vi "Actor Core.vi"(8 "error in":errorcluster, 11 "Basic Demo in":refnum<class "Basic Demo.lvclass">) -> (0 "error out":errorcluster, 3 "Actor out":refnum<class "Actor.lvclass">)   [LabVIEW 2020, in "2. Basic Panel Actors.lvlib" / "Basic Demo.lvclass"]
doc: "Allows the user to launch more panels of different types.\n----\nCopyright: MGI 2016\nAuthor: Derek Trepanier"
uses:
  Basic Demo.lvclass
  C:/Program Files/National Instruments/LabVIEW 2020/vi.lib/MGI/Panel Manager/Panel Actor/Panel Actor/Panel Actor.lvclass
  <vilib>/ActorFramework/Actor/Actor.lvclass
  Panel/Sample Panel.lvclass
  <vilib>/ActorFramework/Message Enqueuer/Message Enqueuer.lvclass
  <vilib>/ActorFramework/Message Enqueuer/Message Enqueuer.lvclass/Message Enqueuer.ctl
  <vilib>/ActorFramework/Message Enqueuer/Enqueue.vi
  Description Panel/Description Panel.lvclass
  <vilib>/MGI/Panel Manager/Panel/Panel/Subpanel/Subpanel.lvclass
  C:/Program Files/National Instruments/LabVIEW 2020/vi.lib/MGI/Panel Manager/Panel/Panel/Panel.lvclass
  <vilib>/ActorFramework/Stop Msg/Stop Msg.lvclass
  C:/Program Files/National Instruments/LabVIEW 2020/vi.lib/ActorFramework/Message/Message.lvclass
  <vilib>/MGI/Panel Manager/Panel/Panel/Window/Dialog/Dialog.lvclass
  <vilib>/MGI/Panel Manager/Panel/Panel/Window/Window.lvclass
  <vilib>/MGI/Panel Manager/Panel/Panel/Subpanel/Subpanel.vi
  <vilib>/ActorFramework/Message Priority Queue/Priority Enqueue.vi
  <vilib>/MGI/Panel Manager/Panel/Panel/Window/Dialog/Dialog.vi
  <vilib>/MGI/Panel Manager/Panel/Panel/Window/Window.vi
  <vilib>/MGI/Panel Manager/Panel Actor/Panel Actor/Panel Actor.lvclass
  <vilib>/MGI/Panel Manager/Panel Actor/Panel Actor Messages/Show Panel Msg/Show Panel Msg.lvclass
  <vilib>/MGI/Panel Manager/Panel/Panel.lvlib
panel:
  in  "Show Window":bool
  in  "Show Dialog":bool
  in  "Running Sub-Panels":i32(listbox)
  in  "New Subpanel Item":bool
  # "Windows"
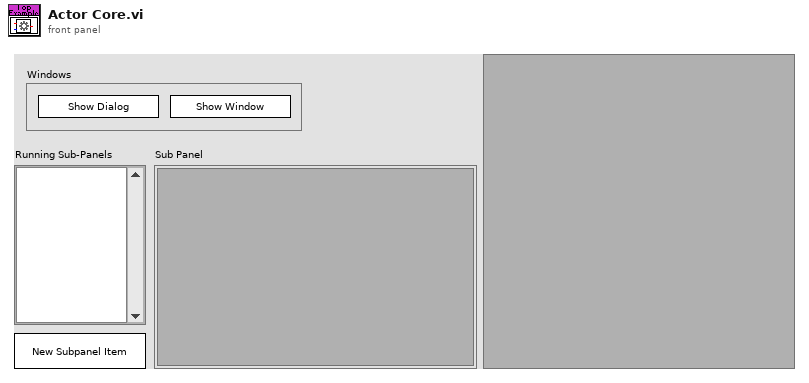
[diagram p1: front panel]
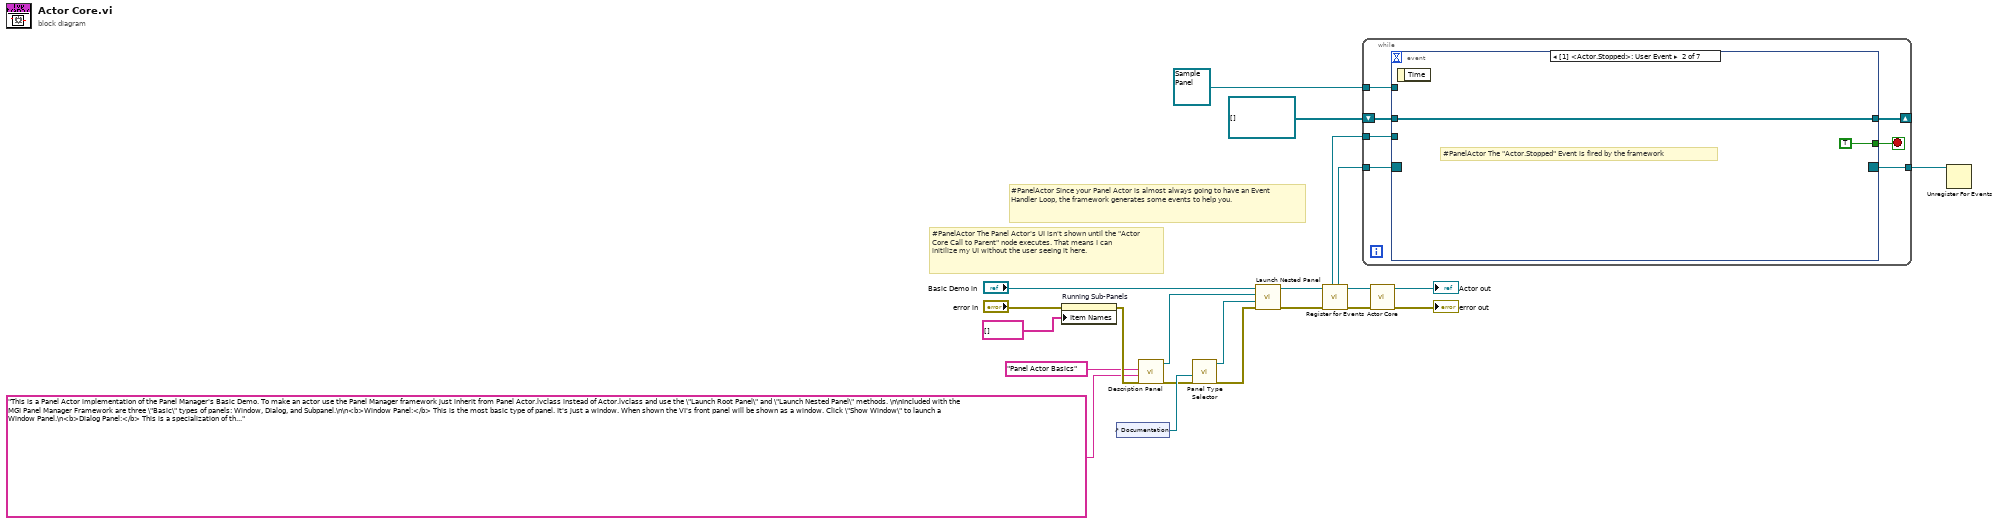
[diagram p0: block diagram]
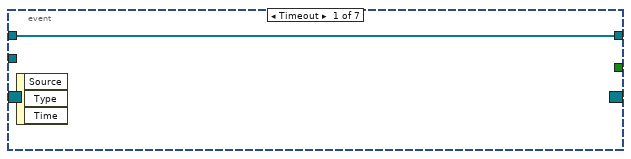
[diagram p2: hidden frame]
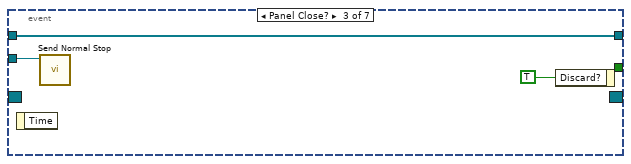
[diagram p3: hidden frame]
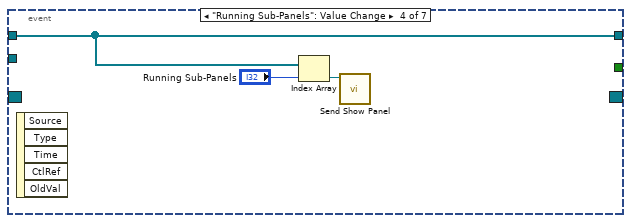
[diagram p4: hidden frame]
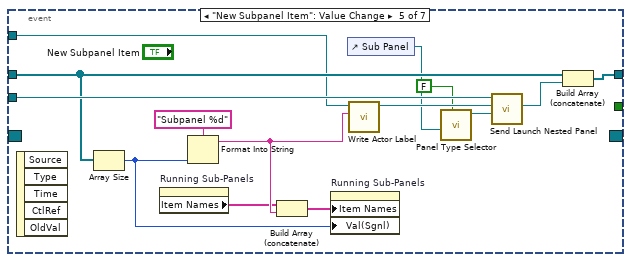
[diagram p5: hidden frame]
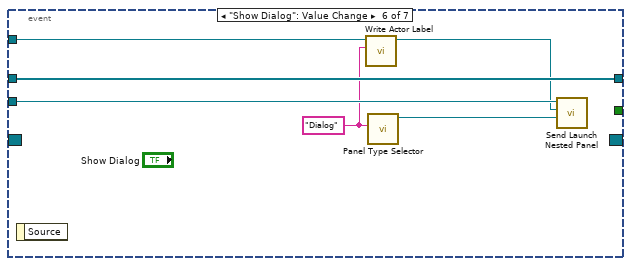
[diagram p6: hidden frame]
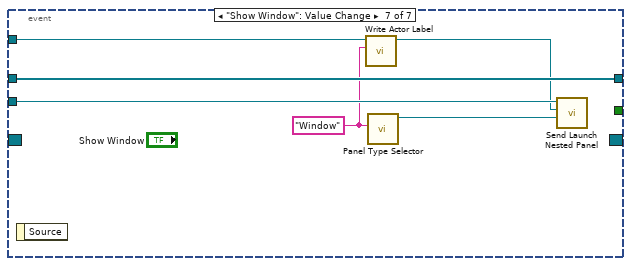
[diagram p7: hidden frame]
diagram:
  # "#PanelActor Since your Panel Actor is almost always going to have an Event Handler Loop, the framework generates some events to help you."
  # "#PanelActor The Panel Actor's UI isn't shown until the \"Actor Core Call to Parent\" node executes. That means I can initilize my UI without the user seeing it here."
  n1 = property on="Running Sub-Panels" class="LstBox (strict)"(error in="error in", "Item Names"=string[] []) -> (error out=w8:errorcluster)  [unwired: 1 in, 1 out]
  n2 = control-ref of="Documentation"() -> (w16:refnum<vi>)
  n3 = call "Description Panel.vi"("error in (no error)"=w8, "Description"="This is a Panel Actor implementation of the Panel Manager's Basic Demo. To make an actor use the Panel Manager framework just inherit from Panel Actor.lvclass instead of Actor.lvclass and use the \"Launch Root Panel\" and \"Launch Nested Panel\" methods. \n\nIncluded with the MGI Panel Manager Framework are three \"Basic\" types of panels: Window, Dialog, and Subpanel.\n\n<b>Window Panel:</b> This is the most basic type of panel. It's just a window. When shown the VI's front panel will be shown as a window. Click \"Show Window\" to launch a Window Panel.\n<b>Dialog Panel:</b> This is a specialization of the window panel. Again, the window will just be shown as a window, but the front panel will be set to modal. Click \"Show Dialog\" to launch a Dialog Panel.\n<b>Subpanel:</b> This panel type will insert the front panel into a subpanel of another VI. Click \"New Subpanel Item\" to launch a new Subpanel Panel. The list of running subpanel items is show in the \"Running Sub-Panels\" \n\nView the #PanelActor bookmark for more info.\n" ("Description Title"), "Description Title"="Panel Actor Basics") -> ("error out"=w7:errorcluster, "Description Panel out"=w4:refnum<class "Description Panel.lvclass">)  [unwired: 7 in]
  n4 = call-poly <vilib>:"Panel Type Selector.vi"("Error In"=w7, "Sub Panel"=w16) -> ("Error Out"=w6:errorcluster, "Subpanel Out"=w5:refnum<class "Subpanel.lvclass">)  [unwired: 8 in]
  n5 = call <vilib>:"Launch Nested Panel.vi"("error in (no error)"=w6, "Panel"=w5, "Nested Panel Actor"=w4, "Panel Actor in"="Basic Demo in") -> ("error out"=w9:errorcluster, "Panel Actor out"=w10:refnum<class "Basic Demo.lvclass">)  [unwired: 4 in, 2 out]
  n6 = call <vilib>:"Register for Events.vi"("Error In"=w9, "Panel Actor in"=w10) -> ("Error Out"=w20:errorcluster, "Panel Actor out"=w21:refnum<class "Basic Demo.lvclass">, "Pnl Actor"=w19:refnum<event-registration>, "Self Enqueuer"=w18:refnum<class "Message Enqueuer.lvclass">)  [unwired: 6 in]
  n7 = while {
    tunnel: w19 -> [w29]
    tunnel: w18 -> [w28]
    shift-right: [w25] -> _
    shift-left: refnum<class "Message Enqueuer.lvclass">[] [] -> [w26]
    tunnel: refnum<class "Sample Panel.lvclass"> refnum ("Basic Panel Actors.lvlib:Panel.lvclass") -> [w24]
    tunnel: [w23] -> w1
    stop <- w27 stop-if-true
    n8 = event shown="[1] <Actor.Stopped>: User Event" {
      selector: w29 -> [_ _ _ _ _ _ _]
      dyn-events: [_ _ _ _ _ _ _] -> w23
      timeout: _ -> [_ _ _ _ _ _ _]
      tunnel: w28 -> [_ _ w34 _ w49 w57 w63]
      tunnel: [_ TRUE _ _ _ _ _] -> w27
      tunnel: w26 -> [w30 w31 w33 w38 w46 w58 w64]
      tunnel: [w30 w31 w33 w38 w52 w58 w64] -> w25
      tunnel: w24 -> [_ _ _ _ w44 w56 w62]
      event Timeout {
        n9 = event-data() -> ()  [unwired: 1 in, 3 out]
      }
      event User Event {
        # "#PanelActor The \"Actor.Stopped\" Event is fired by the framework"
        n10 = event-data() -> ()  [unwired: 1 in, 1 out]
      }
      event Panel Close? {
        n11 = event-data() -> ()  [unwired: 1 in, 1 out]
        n12 = call <vilib>:"Send Normal Stop.vi"("Message Enqueuer"=w34) -> ()  [unwired: 10 in, 1 out]
        n13 = event-data("Discard?"=TRUE) -> ()  [unwired: 1 in, 1 out]
      }
      event "Running Sub-Panels": Value Change {
        n14 = event-data() -> ()  [unwired: 1 in, 5 out]
        n15 = Index Array(array=w38, index="Running Sub-Panels") -> (element=w37:refnum<class "Message Enqueuer.lvclass">)
        n16 = call <vilib>:"Send Show Panel.vi"("Message Enqueuer in"=w37) -> ()  [unwired: 9 in, 2 out]
      }
      event "New Subpanel Item": Value Change {
        n17 = event-data() -> ()  [unwired: 1 in, 5 out]
        n18 = Array Size(array=w46) -> (size(s)=w41:i32)
        n19 = property on="Running Sub-Panels" class="LstBox (strict)"() -> ("Item Names"=w43:string[])  [unwired: 2 in, 2 out]
        n20 = Format Into String(format string="Subpanel %d", w41) -> (resulting string=w45:string)  [unwired: 2 in, 1 out]
        n21 = Build Array (concatenate)(w43, w45) -> (w42:string[])
        n22 = property on="Running Sub-Panels" class="LstBox (strict)"("Item Names"=w42, "Val(Sgnl)"=w41) -> ()  [unwired: 2 in, 2 out]
        n23 = control-ref of="Sub Panel"() -> (w40:refnum<vi>)
        n24 = call-dynamic "Write Actor Label.vi"("Actor Label"=w45, "Monitored Actor in"=w44) -> ("Monitored Actor out"=w48:refnum<class "Sample Panel.lvclass">)  [unwired: 8 in, 1 out]
        n25 = call-poly <vilib>:"Panel Type Selector.vi"("Autoshow? (T)"=FALSE, "Sub Panel"=w40) -> ("Subpanel Out"=w50:refnum<class "Subpanel.lvclass">)  [unwired: 8 in, 1 out]
        n26 = call <vilib>:"Send Launch Nested Panel.vi"("Panel"=w50, "Nested Panel Actor"=w48, "Self Enqueuer in"=w49) -> ("Nested Actor's Enqueuer"=w51:refnum<class "Message Enqueuer.lvclass">)  [unwired: 7 in, 1 out]
        n27 = Build Array (concatenate)(w46, w51) -> (w52:refnum<class "Message Enqueuer.lvclass">[])
      }
      event "Show Dialog": Value Change {
        w53 = "Dialog" ("Title")
        n28 = event-data() -> ()  [unwired: 1 in, 1 out]
        n29 = call-dynamic "Write Actor Label.vi"("Actor Label"=w53, "Monitored Actor in"=w56) -> ("Monitored Actor out"=w54:refnum<class "Sample Panel.lvclass">)  [unwired: 8 in, 1 out]
        n30 = call-poly <vilib>:"Panel Type Selector.vi"("Default Title"=w53) -> ("Dialog out"=w55:refnum<class "Dialog.lvclass">)  [unwired: 9 in, 1 out]
        n31 = call <vilib>:"Send Launch Nested Panel.vi"("Panel"=w55, "Nested Panel Actor"=w54, "Self Enqueuer in"=w57) -> ()  [unwired: 7 in, 2 out]
      }
      event "Show Window": Value Change {
        w59 = "Window" ("Title")
        n32 = event-data() -> ()  [unwired: 1 in, 1 out]
        n33 = call-dynamic "Write Actor Label.vi"("Actor Label"=w59, "Monitored Actor in"=w62) -> ("Monitored Actor out"=w60:refnum<class "Sample Panel.lvclass">)  [unwired: 8 in, 1 out]
        n34 = call-poly <vilib>:"Panel Type Selector.vi"("Default Title"=w59) -> ("Window out"=w61:refnum<class "Window.lvclass">)  [unwired: 9 in, 1 out]
        n35 = call <vilib>:"Send Launch Nested Panel.vi"("Panel"=w61, "Nested Panel Actor"=w60, "Self Enqueuer in"=w63) -> ()  [unwired: 7 in, 2 out]
      }
    }
  }
  n36 = call-parent "Actor Core.vi"("error in"=w20, "Panel Actor in"=w21) -> ("error out"=→"error out":errorcluster, "Actor out"=→"Actor out":refnum<class "Actor.lvclass">)  [unwired: 8 in]
  n37 = Unregister For Events(event registration refnum=w1) -> ()  [unwired: 1 in, 1 out]
